vi "Interpolation Solver_dataviewer.vi"(7 "method":T2(ring)=enum."Spline", 9 "factor":i32=11, 10 "x-original":dbl[](array[numeric])=[0.0, 1.2, 2.0, 3.0, 3.5, 4.0, 5.0], 11 "y-original":dbl[](array[numeric])=[1.0, 2.700000047683716, 7.400000095367432, 150.0, 140.0, 80.0, 220.0]) -> (2 "x-interpolated":dbl[](array[numeric]), 3 "y-interpolated":dbl[](array[numeric]))   [LabVIEW 2021]
doc: "Demonstrates different types of interpolation on a set of raw data. The types of interpolation demonstrated in this example are Linear, Polynomial, Spline, and Rational."
uses:
  <vilib>/Analysis/NI_AALPro.lvlib
panel:
  out "error out":errorcluster
  out "Raw and Interpolated Data":T1(graph)=[{"Original Data (X,Y)"=[0.0, 1.2, 2.0, 3.0, 3.5, 4.0, 5.0], "Original Data (X,Y)"=[1.0, 2.700000047683716, 7.400000095367432, 150.0, 140.0, 80.0, 220.0]}, {"Original Data (X,Y)"=[0.0, 0.09999999999999999, 0.19999999999999998, 0.3, 0.39999999999999997, 0.5, 0.6, 0.7000000000000001, 0.7999999999999999, 0.8999999999999999, 1.0, 1.0999999999999999, 1.2, 1.2666666666666666, 1.3333333333333333, 1.4, 1.4666666666666666, 1.5333333333333334, 1.6, 1.6666666666666665, 1.7333333333333334, 1.8, 1.8666666666666667, 1.9333333333333333, 2.0, 2.0833333333333335, 2.1666666666666665, 2.25, 2.3333333333333335, 2.4166666666666665, 2.5, 2.5833333333333335, 2.6666666666666665, 2.75, 2.8333333333333335, 2.9166666666666665, 3.0, 3.041666666666667, 3.083333333333333, 3.125, 3.166666666666667, 3.208333333333333, 3.25, 3.291666666666667, 3.333333333333333, 3.375, 3.416666666666667, 3.458333333333333, 3.5, 3.5416666666666665, 3.5833333333333335, 3.625, 3.6666666666666665, 3.7083333333333335, 3.75, 3.7916666666666665, 3.8333333333333335, 3.875, 3.9166666666666665, 3.9583333333333335, 4.0, 4.083333333333333, 4.166666666666667, 4.25, 4.333333333333333, 4.416666666666667, 4.5, 4.583333333333333, 4.666666666666667, 4.75, 4.833333333333333, 4.916666666666667, 5.0], "Original Data (X,Y)"=[1.0, 2.3924029604023143, 3.732327475080349, 4.967295098309824, 6.044827384366458, 6.912445887525974, 7.5176721620640885, 7.8080277622565255, 7.7310342423790015, 7.23421315670724, 6.265086059516957, 4.771174505083877, 2.700000047683716, 1.000579506543195, -0.82639929721429, -2.628609582342879, -4.253724567596707, -5.549417471729917, -6.363361513496636, -6.54322991165102, -5.936695884947188, -4.3914326521392875, -1.755113431981461, 2.124588556772159, 7.400000095367432, 16.068903365453245, 26.733298416919904, 38.96987026382418, 52.35530392022265, 66.46628440017192, 80.87949671772876, 95.17162588694978, 108.91935692189152, 121.69937483661082, 133.08836464516423, 142.66301136160837, 150.0, 152.7067362173637, 154.75321245875486, 156.1444120142, 156.8853181737255, 156.9809142273579, 156.43618346512363, 155.25610917704915, 153.44567465316098, 151.0098631834855, 147.95365805804917, 144.28204256687857, 140.0, 135.13403211106163, 129.7967145081979, 124.12214126316489, 118.24440644771866, 112.2976041336152, 106.41582839261069, 100.73317329646115, 95.38373291692258, 90.50160132575115, 86.22087259470287, 82.67564079553378, 80.0, 77.5593153292216, 78.79880926821149, 83.38392012517251, 90.98008620830757, 101.25274582581966, 113.86733728591145, 128.48929889678593, 144.78406896664615, 162.41708580369465, 181.0537877161345, 200.3596130121688, 220.0]}]
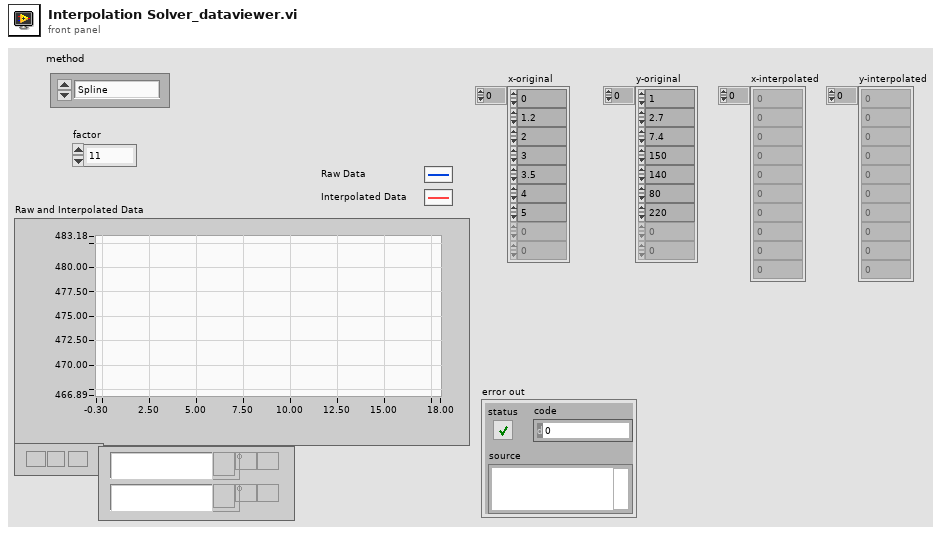
[diagram p1: front panel]
types:
  T1 = cluster{"Original Data (X,Y)":dbl[], "Original Data (X,Y)":dbl[]}[]
  T2 = enum16{"Linear", "Polynomial", "Spline", "Rational"}
  T3 = cluster{"x-original":dbl[], "y-original":dbl[]}[]
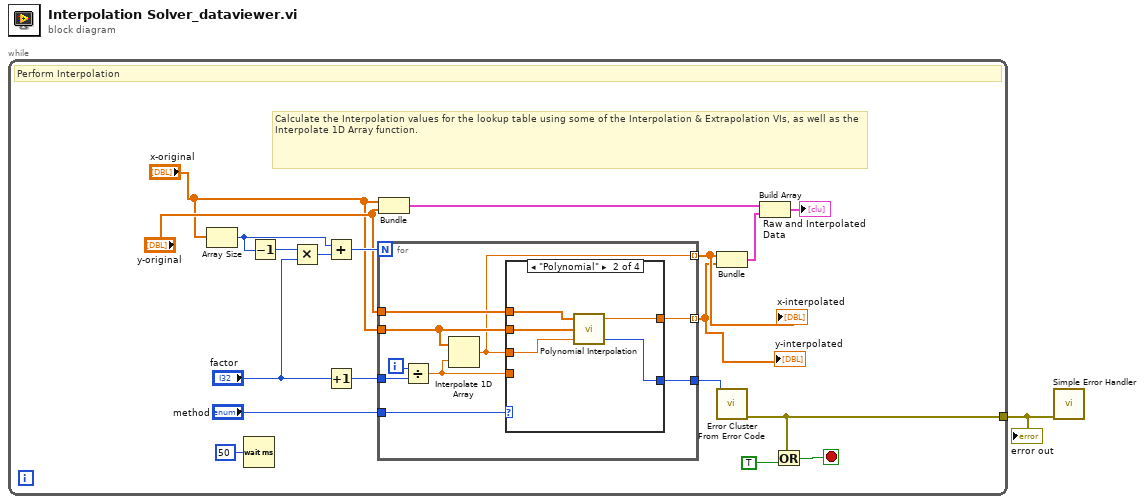
[diagram p0: block diagram]
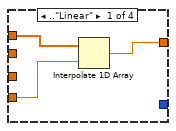
[diagram p2: hidden frame]
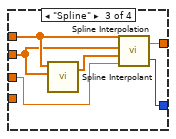
[diagram p3: hidden frame]
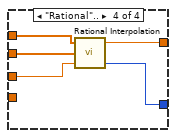
[diagram p4: hidden frame]
diagram:
  n1 = while {
    tunnel: [w6] -> w1
    stop <- w7 stop-if-true
    # "Calculate the Interpolation values for the lookup table using some of the Interpolation & Extrapolation VIs, as well as the Interpolate 1D Array function."
    # "Perform Interpolation"
    n2 = Array Size(array="x-original") -> (size(s)=w12:i32)
    n3 = Wait (ms)(milliseconds to wait=u32 50) -> ()  [unwired: 1 out]
    n4 = Decrement(x=w12) -> (x-1=w15:i32)
    n5 = Multiply(x=w15, y="factor") -> (x*y=w13:i32)
    n6 = Add(x=w12, y=w13) -> (x+y=w11:i32)
    n7 = Increment(x="factor") -> (x+1=w14:i32)
    n8 = for {
      N: w11 -> [_]
      tunnel: "y-original" -> [w29]
      tunnel: "x-original" -> [w23]
      tunnel: [w28] -> w8
      tunnel: "method" -> [w24]
      tunnel: w14 -> [w26]
      tunnel: [w25] -> w4 mode=indexing
      tunnel: [w22] -> w5 mode=indexing
      i -> [w27]
      n9 = Divide(x=w27, y=w26) -> (x/y=w21:dbl)
      n10 = Interpolate 1D Array(1:w21, 2:w23) -> (0:w22:dbl)
      n11 = case shown="\"Polynomial\"" w24 {
        tunnel: w22 -> [_ w37 w40 w44]
        tunnel: [w31 w36 w38 w46] -> w25
        tunnel: [_ w35 w39 w45] -> w28
        tunnel: w23 -> [_ w34 w41 w47]
        tunnel: w29 -> [w32 w33 w43 w48]
        tunnel: w21 -> [w30 _ _ _]
        frame .."Linear" {
          n12 = Interpolate 1D Array(1:w30, 2:w32) -> (0:w31:dbl)
        }
        frame "Polynomial" {
          n13 = call <vilib>:"Polynomial Interpolation.vi"("x value"=w37, "X"=w34, "Y"=w33) -> ("error"=w35:i32, "interpolation value"=w36:dbl)  [unwired: 1 out]
        }
        frame "Spline" {
          n14 = call <vilib>:"Spline Interpolant.vi"("X"=w41, "Y"=w43) -> ("Interpolant"=w42:dbl[])  [unwired: 2 in, 1 out]
          n15 = call <vilib>:"Spline Interpolation.vi"("x value"=w40, "Interpolant"=w42, "X"=w41, "Y"=w43) -> ("error"=w39:i32, "interpolation value"=w38:dbl)
        }
        frame "Rational".. {
          n16 = call <vilib>:"Rational Interpolation.vi"("x value"=w44, "X"=w47, "Y"=w48) -> ("error"=w45:i32, "interpolation value"=w46:dbl)  [unwired: 1 out]
        }
      }
    }
    "x-interpolated" <- w5
    "y-interpolated" <- w4
    n17 = Bundle("x-original"="x-original", "y-original"="y-original") -> (w16:cluster{"x-original":dbl[], "y-original":dbl[]})  [unwired: 1 in]
    n18 = Bundle(w5, w4) -> (w17:cluster{dbl[], dbl[]})  [unwired: 1 in]
    n19 = call <vilib>:"Error Cluster From Error Code.vi"("error code (0)"=w8) -> ("error out"=w6:errorcluster)  [unwired: 8 in]
    n20 = Build Array(w16, w17) -> (→"Raw and Interpolated Data":T3)
    n21 = Or(x=w6, y=TRUE) -> (x .or. y?=w7:bool)
  }
  "error out" <- w1
  n22 = call <vilib>:"Simple Error Handler.vi"("error in (no error)"=w1) -> ()  [unwired: 4 in, 5 out]
